vi "Create Request Description.vi"(8 "error in (no error)":errorcluster, 10 "JSON in":string, 11 "Help in":refnum<class "Help.lvclass">) -> (0 "error out":errorcluster, 2 "<JSON> out":string, 3 "Help out":refnum<class "Help.lvclass">)   [LabVIEW 2019, in "Instrument.lvlib" / "Help.lvclass"]
uses:
  Help.lvclass
  Help.lvclass/Help.ctl
  <vilib>/ciozi137/JSON-Schema/API/Read Typedef Description (variant).vi
  <vilib>/JDP Science/JSONtext/JSONtext.lvlib
  <vilib>/ciozi137/JSON-Schema/JSON-Schema.lvlib
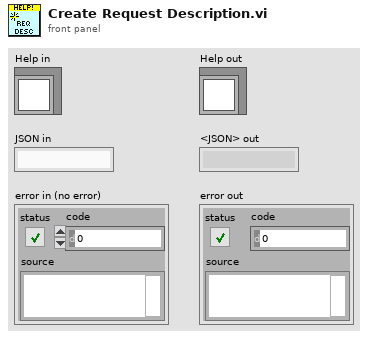
[diagram p1: front panel]
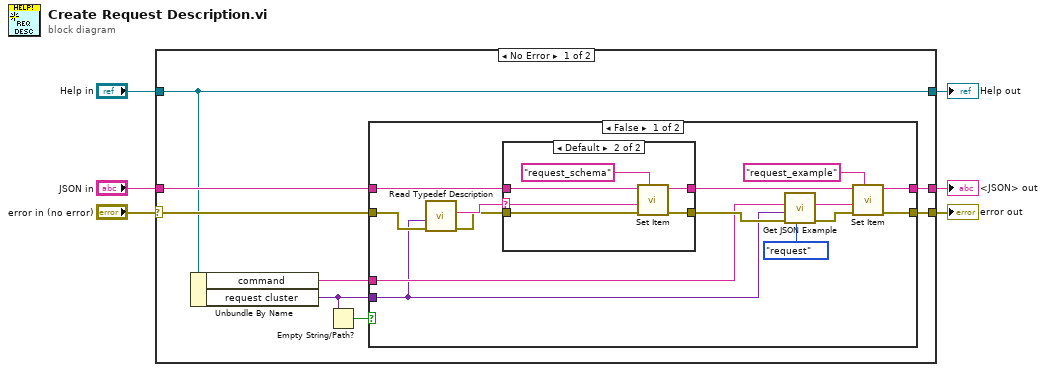
[diagram p0: block diagram]
diagram:
  n1 = case shown="No Error" "error in (no error)" {
    selector: "error in (no error)" -> [w8 w40]
    tunnel: "JSON in" -> [w14 w39]
    tunnel: [w11 w39] -> w4
    tunnel: [w10 w40] -> w5
    tunnel: "Help in" -> [w7 w41]
    tunnel: [w7 w41] -> w1
    frame No Error {
      n2 = Unbundle By Name(w7) -> ("command"=w13:string, "request cluster"=w9:variant)
      n3 = Empty String/Path?(string/path=w9) -> (empty?=w12:bool)
      n4 = case shown="False" w12 {
        tunnel: w14 -> [w28 w38]
        tunnel: w13 -> [w25 _]
        tunnel: [w24 w38] -> w11
        tunnel: [w23 w37] -> w10
        tunnel: w9 -> [w15 _]
        tunnel: w8 -> [w17 w37]
        frame False {
          n5 = call-poly <vilib>:"Read Typedef Description.vi"("error in (no error)"=w17, "variant"=w15) -> ("error out"=w16:errorcluster, "VI description"=w22:string)  [unwired: 7 in, 1 out]
          n6 = case shown="Default" w22 {
            selector: w22 -> [_ w34]
            tunnel: w28 -> [w30 w36]
            tunnel: w16 -> [w29 w35]
            tunnel: [w30 w33] -> w27
            tunnel: [w29 w32] -> w26
            frame "", "{}" {
            }
            frame Default {
              n7 = call <vilib>:"Set Item.vi"("$Path or Item Name"="request_schema", "error in (no error)"=w35, "JSON to Insert"=w34, "JSON"=w36) -> ("error out"=w32:errorcluster, "<JSON>"=w33:string)  [unwired: 4 in, 1 out]
            }
          }
          n8 = call "Get JSON Example.vi"("type"=enum16{"request", "response"}."request", "error in (no error)"=w26, "params or result"=w15, "method"=w25) -> ("error out"=w19:errorcluster, "<JSON>"=w20:string)  [unwired: 6 in]
          n9 = call <vilib>:"Set Item.vi"("$Path or Item Name"="request_example", "error in (no error)"=w19, "JSON to Insert"=w20, "JSON"=w27) -> ("error out"=w23:errorcluster, "<JSON>"=w24:string)  [unwired: 4 in, 1 out]
        }
        frame True {
        }
      }
    }
    frame Error {
    }
  }
  "Help out" <- w1
  "error out" <- w5
  "<JSON> out" <- w4
